vi "RunVI.vi"(8 "error in (no error)":errorcluster, 10 "machine name (\"\":  open local reference)":string, 11 "String":string) -> (0 "error out":errorcluster)   [LabVIEW 2021]
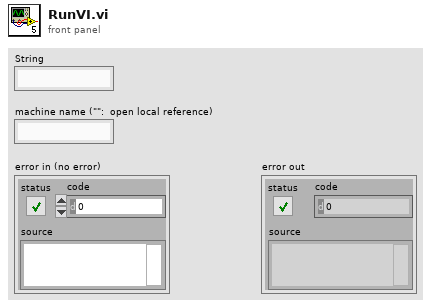
[diagram p1: front panel]
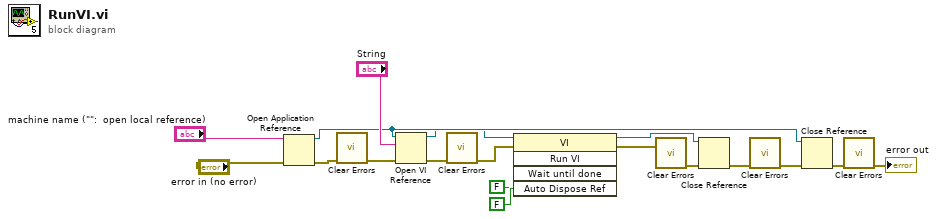
[diagram p0: block diagram]
diagram:
  n1 = Open Application Reference(8:"error in (no error)", 11:"machine name (\"\":  open local reference)") -> (0:w9:errorcluster, 3:w7:refnum<vi>)  [unwired: 2 in]
  n2 = call <vilib>:"Clear Errors.vi"("error in (no error)"=w9) -> ("error out"=w10:errorcluster)  [unwired: 5 in, 1 out]
  n3 = Open VI Reference(application reference (local)=w7, vi path="String", error in (no error)=w10) -> (vi reference=w3:refnum<vi>, error out=w11:errorcluster)  [unwired: 3 in]
  n4 = call <vilib>:"Clear Errors.vi"("error in (no error)"=w11) -> ("error out"=w12:errorcluster)  [unwired: 5 in, 1 out]
  n5 = invoke class="VI" method="Run VI"(reference=w3, error in=w12, "Wait until done"=FALSE ("Wait Until Done"), "Auto Dispose Ref"=FALSE ("Auto Dispose Reference")) -> (reference out=w6:refnum<vi>, error out=w13:errorcluster)  [unwired: 1 in, 3 out]
  n6 = call <vilib>:"Clear Errors.vi"("error in (no error)"=w13) -> ("error out"=w14:errorcluster)  [unwired: 5 in, 1 out]
  n7 = Close Reference(reference=w6, error in (no error)=w14) -> (error out=w15:errorcluster)
  n8 = call <vilib>:"Clear Errors.vi"("error in (no error)"=w15) -> ("error out"=w16:errorcluster)  [unwired: 5 in, 1 out]
  n9 = Close Reference(reference=w7, error in (no error)=w16) -> (error out=w17:errorcluster)
  n10 = call <vilib>:"Clear Errors.vi"("error in (no error)"=w17) -> ("error out"=→"error out":errorcluster)  [unwired: 5 in, 1 out]
